vi "WaitAnswer.vi"(1 "VISA resource name in":refnum<visa-resource-name>) -> (0 "VISA resource name out":refnum<visa-resource-name>)   [LabVIEW 2014]
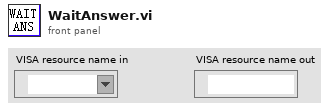
[diagram p1: front panel]
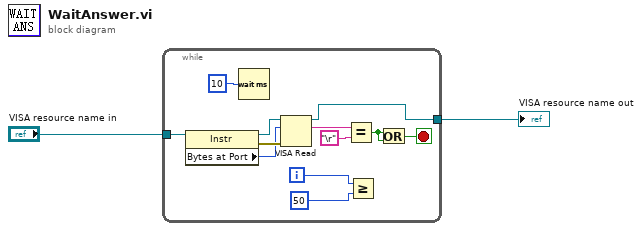
[diagram p0: block diagram]
diagram:
  n1 = while {
    tunnel: "VISA resource name in" -> [w9]
    tunnel: [w4] -> w1
    i -> [w13]
    stop <- w7 stop-if-true
    n2 = property class="Instr"(reference=w9) -> (reference out=w11:refnum<visa-resource-name>, error out=w10:errorcluster, "Bytes at Port"=w8:u32)  [unwired: 1 in]
    n3 = Wait (ms)(milliseconds to wait=u32 10 ("等待时间（毫秒）")) -> ()  [unwired: 1 out]
    n4 = VISA Read(VISA resource name=w11, byte count=w8, error in (no error)=w10) -> (VISA resource name out=w4:refnum<visa-resource-name>, read buffer=w6:string)  [unwired: 2 out]
    n5 = Equal?(x=w6, y="\r") -> (x = y?=w3:bool)
    n6 = Greater Or Equal?(x=w13, y=50) -> ()  [unwired: 1 out]
    n7 = Or(x=w3, y=w3) -> (x .or. y?=w7:bool)
  }
  "VISA resource name out" <- w1
